vi "Filter String.vi"(1 "Index":i32, 2 "String In":string) -> (0 "String Out":string)   [LabVIEW 2025]
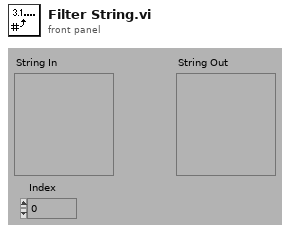
[diagram p1: front panel]
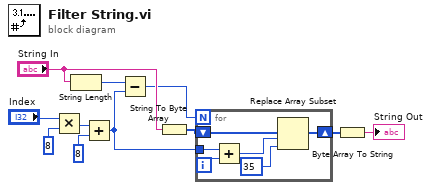
[diagram p0: block diagram]
diagram:
  n1 = Multiply(x="Index", y=8 ("digit")) -> (x*y=w2:i32)
  n2 = String Length(string="String In") -> (length=w11:i32)
  n3 = Add(x=w2, y=8 ("digit")) -> (x+y=w1:i32)
  n4 = Subtract(x=w11, y=w1) -> (x-y=w6:i32)
  n5 = String To Byte Array(string="String In") -> (unsigned byte array=w7:u8[])
  n6 = for {
    N: w6 -> [_]
    shift-right: [w16] -> w9
    shift-left: w7 -> [w15]
    tunnel: w1 -> [w14]
    i -> [w13]
    n7 = Add(x=w14, y=w13) -> (x+y=w12:i32)
    n8 = Replace Array Subset(array=w15, new element=u8 35, index=w12) -> (w16:u8[])
  }
  n9 = Byte Array To String(unsigned byte array=w9) -> (string=→"String Out":string)
